vi "Open.vi"(8 "Error In":errorcluster, 11 "Omega CSi32 In":refnum<visa-resource-name>) -> (0 "Error Out":errorcluster, 3 "Omega CSi32 Out":refnum<visa-resource-name>)   [LabVIEW 2012, in "Omega-CSi32.lvlib"]
uses:
  Omega-CSi32.lvlib
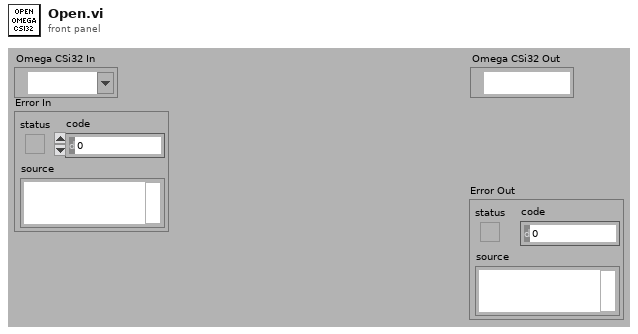
[diagram p1: front panel]
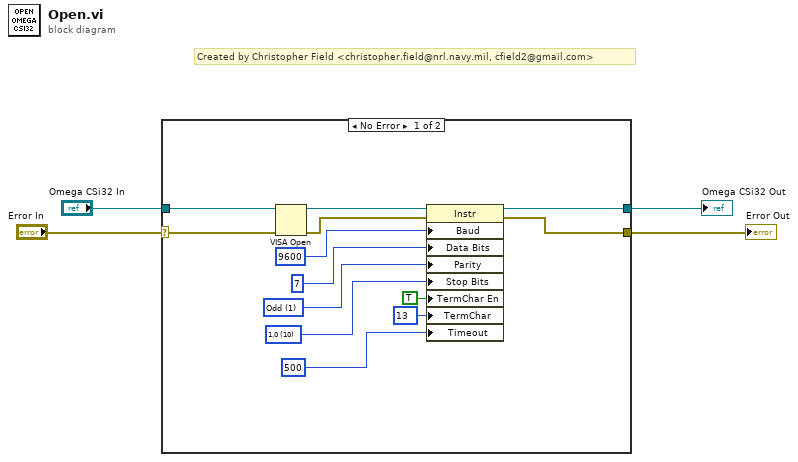
[diagram p0: block diagram]
diagram:
  # "Created by Christopher Field <christopher.field@nrl.navy.mil, cfield2@gmail.com>"
  n1 = case shown="No Error" "Error In" {
    selector: "Error In" -> [w5 w18]
    tunnel: "Omega CSi32 In" -> [w17 w19]
    tunnel: [w10 w19] -> w3
    tunnel: [w9 w18] -> w2
    frame No Error {
      w11 = u16 10 items=["1.0"=10, "1.5"=15, "2.0"=20] ("Serial Settings:Stop Bits")
      w12 = u16 1 items=["None", "Odd", "Even", "Mark", "Space"] ("Serial Settings:Parity")
      n2 = VISA Open(error in (no error)=w5, VISA resource name=w17) -> (VISA resource name=w16:refnum<visa-resource-name>, error out=w14:errorcluster)  [unwired: 3 in]
      n3 = property class="Instr"(reference=w16, error in=w14, "Baud"=u32 9600 ("Serial Settings:Baud Rate"), "Data Bits"=u16 7 ("Serial Settings:Data Bits"), "Parity"=w12, "Stop Bits"=w11, "TermChar En"=TRUE ("Message Based Settings:Termination Character Enable"), "TermChar"=u8 13 ("Message Based Settings:Termination Character"), "Timeout"=u32 500 ("General Settings:Timeout Value")) -> (reference out=w10:refnum<visa-resource-name>, error out=w9:errorcluster)
    }
    frame Error {
    }
  }
  "Omega CSi32 Out" <- w3
  "Error Out" <- w2
